vi "Tab-Control-With-Password-Protecting.vi"() -> ()   [LabVIEW 2014]
panel:
  in  "stop":bool
  in  "Tab Control":enum32{"Home", "Config"}(tab)
  out "My Secret":string
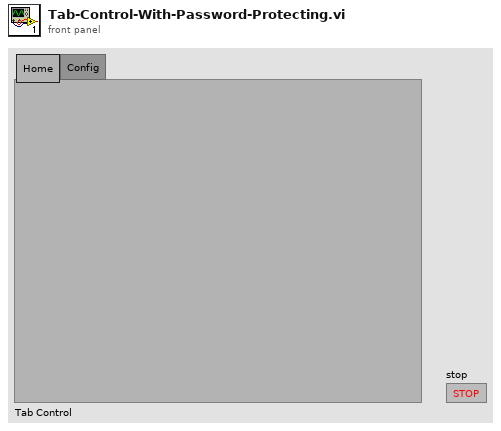
[diagram p1: front panel]
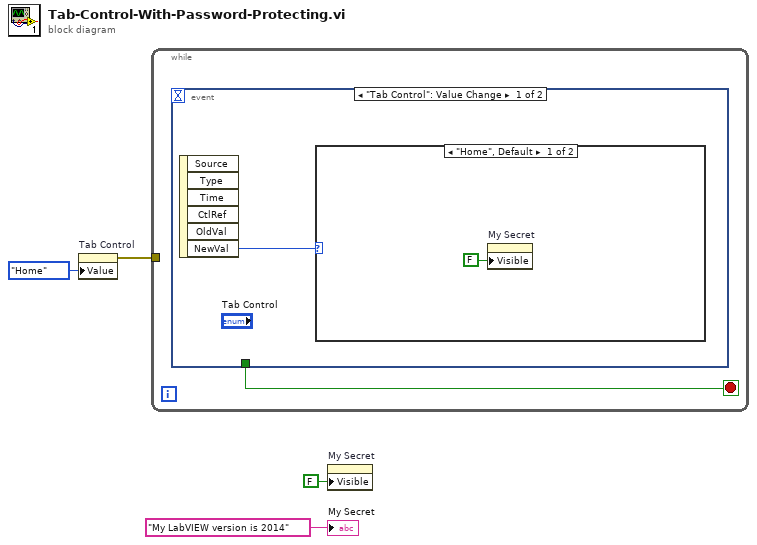
[diagram p0: block diagram]
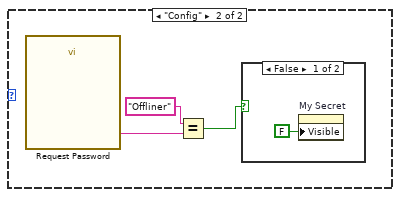
[diagram p2: hidden frame]
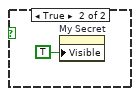
[diagram p3: hidden frame]
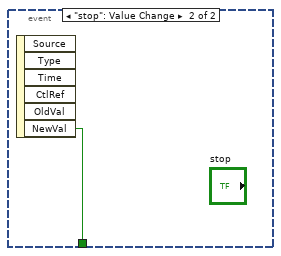
[diagram p4: hidden frame]
diagram:
  n1 = property on="Tab Control" class="TabCtl (strict)"("Value"=enum32{"Home", "Config"}."Home" ("Tab Control")) -> (error out=w4:errorcluster)  [unwired: 2 in, 1 out]
  n2 = while {
    tunnel: w4 -> [_]
    stop <- w5 stop-if-true
    n3 = event shown="[0] \"Tab Control\": Value Change" {
      selector: _ -> [_ _]
      dyn-events: _ -> [_ _]
      timeout: _ -> [_ _]
      tunnel: [_ w13] -> w5
      event "Tab Control": Value Change {
        n4 = event-data() -> ("NewVal"=w6:enum32{"Home", "Config"})  [unwired: 1 in, 5 out]
        n5 = case shown="\"Home\", Default" w6 {
          frame "Home", Default {
            n6 = property on="My Secret" class="Str"("Visible"=FALSE) -> ()  [unwired: 2 in, 2 out]
          }
          frame "Config" {
            n7 = call "Request Password"() -> ("Password"=w10:string)  [unwired: 17 in, 2 out]
            n8 = Equal?(x="Offliner", y=w10) -> (x = y?=w8:bool)
            n9 = case shown="False" w8 {
              frame False {
                n10 = property on="My Secret" class="Str"("Visible"=FALSE) -> ()  [unwired: 2 in, 2 out]
              }
              frame True {
                n11 = property on="My Secret" class="Str"("Visible"=TRUE) -> ()  [unwired: 2 in, 2 out]
              }
            }
          }
        }
      }
      event "stop": Value Change {
        n12 = event-data() -> ("NewVal"=w13:bool)  [unwired: 1 in, 5 out]
      }
    }
  }
  n13 = property on="My Secret" class="Str"("Visible"=FALSE) -> ()  [unwired: 2 in, 2 out]
  "My Secret" <- "My LabVIEW version is 2014"
